vi "GUI.vi"() -> ()   [LabVIEW 2016]
uses:
  <vilib>/NI/Current Value Table/Type Defs/File Format.ctl
  <vilib>/NI/Current Value Table/Type Defs/Single Tag.ctl
  <vilib>/NI/Current Value Table/Type Defs/Data Types.ctl
  <vilib>/NI/Current Value Table/Type Defs/Tag Grouping set.ctl
  <vilib>/NI/Current Value Table/DataTypes/Boolean_Write.vi
  <vilib>/NI/Current Value Table/DataTypes/Boolean_Read.vi
  <vilib>/NI/Current Value Table/DataTypes/U16_Read.vi
  <vilib>/NI/Current Value Table/DataTypes/U16_Write.vi
  <vilib>/NI/Current Value Table/Type to Enum.vi
  <vilib>/NI/Current Value Table/DataTypes/Boolean_Type To Enum.vi
  <vilib>/NI/Current Value Table/DataTypes/U16_Type To Enum.vi
  MB_Master_Serial.lvclass
  C:/Users/PRANAV/Desktop/Modbus_Scada_Main/Modbus_Scada/MB_Master/MB_Master.lvclass
  <vilib>/NI/Current Value Table/FGVs/CVT Globals.vi
  <vilib>/NI/Current Value Table/FGVs/Tag Memory.vi
  <vilib>/NI/Current Value Table/Memory Block.vi
  <vilib>/NI/Current Value Table/DataTypes/Boolean_Memory Block.vi
  <vilib>/NI/Current Value Table/DataTypes/U16_Memory Block.vi
  <vilib>/NI/Current Value Table/Current Value Table.lvlib
  MB Master.lvlib
panel:
  out "Value_O2 3":u16
  out "Value_N2 3":u16
  out "Vel_Value 3":u16
  out "N2 Gas Pressure 1_Value 3":u16
  out "Temp_Min 4":u16
  out "Hum_Value  3":u16
  out "Value_O2 2":u16
  out "Value_N2 2":u16
  out "Vel_Value 2":u16
  out "N2 Gas Pressure 1_Value 2":u16
  out "Temp_Min 3":u16
  out "Hum_Value  2":u16
  out "Max_O2 2":u16
  out "Max_N2 2":u16
  out "Vel_Max 2":u16
  out "N2 Gas Pressure 1_Max 2":u16
  out "Temp_Max 2":u16
  out "Hum_Max 2":u16
  out "Min_O2 2":u16
  out "Min_N2 2":u16
  out "Vel_Min 2":u16
  out "N2 Gas Pressure 1_Min 2":u16
  out "Temp_Min 5":u16
  out "Hum_Min 2":u16
  out "Value_O2":u16
  out "Value_N2":u16
  out "Vel_Value":u16
  out "N2 Gas Pressure 1_Value":u16
  out "Temp_Min":u16
  out "Hum_Value":u16
  out "Spare AI-1_Value":u16
  out "Spare AI-2_Value":u16
  out "Max_O2":u16
  out "Max_N2":u16
  out "Vel_Max":u16
  out "N2 Gas Pressure 1_Max":u16
  out "Temp_Max":u16
  out "Hum_Max":u16
  out "Spare AI-1_Max":u16
  out "Spare AI-2_Max":u16
  out "Min_O2":u16
  out "Min_N2":u16
  out "Vel_Min":u16
  out "N2 Gas Pressure 1_Min":u16
  out "Temp_Min 2":u16
  out "Hum_Min":u16
  out "Spare AI-1_Min":u16
  out "Spare AI-2_Min":u16
  out "Value_8":bool
  out "Value_9":bool
  out "Value_10":bool
  out "Value_11":bool
  out "Value_12":bool
  out "Value_13":bool
  out "Value_14":bool
  out "Value_1":bool
  out "Value_2":bool
  out "Value_3":bool
  out "Value_4":bool
  out "Value_5":bool
  out "Value_6":bool
  out "Value_7":bool
  out "O.T. Entrance -Cap Proxy":bool
  out "Main Entrance E-stop PB":bool
  out "Doctors Entrance Door-2 Open Proxy FB":bool
  out "Main Entrance Door Open Inside PB":bool
  out "Main Entrance Door Open Proxy FB":bool
  out "O.T Entrance-Nose Mask Proxy":bool
  out "Doctors Entrance Door-1 Open PB":bool
  out "Doctors Entrance Door-1 Open Inside PB":bool
  out "Doctors Entrance Door-1 Open Proxy FB":bool
  out "Doctors Entrance-Nose Mask Proxy":bool
  out "Doctors Entrance-Cap Proxy":bool
  out "Doctors Entrance-Hand Sanitizer  Proxy":bool
  out "Doctors Entrance Door-2 Open Inside PB":bool
  out "Ist O.T.-Occupied Lamp Green":bool
  out "Ist O.T-AHU Start Coil":bool
  out "2nd O.T.:Scrubber Dispense Coil":bool
  out "2nd O.T.-Door Open Cmd":bool
  out "Spare DO-1":bool
  out "Spare DO-2":bool
  out "Spare DO-3":bool
  out "Spare DO-4":bool
  out "Spare DO-5":bool
  out "Spare DO-6":bool
  out "Doctor Entrance Door-1 Open Cmd":bool
  out "Doctor Entrance -Door-2 Open Cmd":bool
  out "Doctor Entrance -Hand Santizier Coil":bool
  out "Main Entrance-Door Open Cmd":bool
  out "OT Entrance-Door Open  Cmd":bool
  out "O.T Entrance-Hand Santiizier Coil":bool
  out "Ist O.T.- Door Open Cmd":bool
  out "Ist O.T-Occupied Lamp(Red)":bool
  out "Ist O.T-Inside Light":bool
  out "Ist O.T.-Scrubber Dispense Coil":bool
  out "error out":errorcluster
  in  "stop  5":bool
  in  "stop  4":bool
  in  "stop  3":bool
  in  "stop  2":bool
  in  "stop":bool
  # "DOORS &\n                    STATUS"
  # "Description"
  # "Status"
  # "Description"
  # "Status"
  # "Doctor Entrance Door-1 Open Cmd"
  # "Ist O.T.-Occupied Lamp Green"
  # "Doctor Entrance -Door-2 Open Cmd"
  # "Ist O.T-AHU Start Coil"
  # "Doctor Entrance -Hand Santizier Coil"
  # "2nd O.T.:Scrubber Dispense Coil"
  # "Main Entrance-Door Open Cmd"
  # "2nd O.T.-Door Open Cmd"
  # "OT Entrance-Door Open  Cmd"
  # "Spare DO-1"
  # "O.T Entrance-Hand Santiizier Coil"
  # "Spare DO-2"
  # "Ist O.T.- Door Open Cmd"
  # "Spare DO-3"
  # "Ist O.T-Occupied Lamp(Red)"
  # "Spare DO-4"
  # "Ist O.T-Inside Light"
  # "Spare DO-5"
  # "Ist O.T.-Scrubber Dispense Coil"
  # "Spare DO-6"
  # "DOORS FB AND SENSOR\n                                  STATUS"
  # "Description"
  # "Status"
  # "Description"
  # "Status"
  # "Doctors Entrance Door-1 Open PB"
  # "Doctors Entrance Door-2 Open Proxy FB"
  # "Doctors Entrance Door-1 Open Inside PB"
  # "Main Entrance E-stop PB"
  # "Doctors Entrance Door-1 Open Proxy FB"
  # "Main Entrance-Strecther Entry PB"
  # "Doctors Entrance-Nose Mask Proxy"
  # "Main Entrance Door Open Inside PB"
  # "Doctors Entrance-Cap Proxy"
  # "Main Entrance Door Open Proxy FB"
  # "Doctors Entrance-Hand Sanitizer  Proxy"
  # "O.T Entrance-Nose Mask Proxy"
  # "Doctors Entrance Door-2 Open Inside PB"
  # "O.T. Entrance -Cap Proxy"
  # "DOORS FB AND SENSOR\n                                  STATUS"
  # "Description"
  # "Status"
  # "Description"
  # "Status"
  # "OT Entrance-Hand Santizier Proxy"
  # "Spare DI-2"
  # "Spare DI-1"
  # "Ist O.T-AHU Run FB"
  # "OT Entrance-Door Inside Open PB"
  # "2nd O.T-Scrubber Proxy"
  # "OT Entrance-Door Open Proxy FB"
  # "2nd O.T-Door Inside Open PB"
  # "Ist O.T -Scrubber Proxy"
  # "2nd O.T-Door Open Proxy FB"
  # "Ist O.T-Door Inside Open PB"
  # "Ist O.T-E-Stop PB"
  # "Ist O.T-Door  Open Proxy FB"
  # "2nd O.T-E-Stop PB"
  # "O.T Parameters"
  # "Description"
  # "Min"
  # "Max"
  # "Value"
  # "Unit"
  # "O2 Gas Pressure"
  # "Bar"
  # "N2 Gas Pressure 1"
  # "Bar"
  # "Velocity"
  # "ft/m"
  # "N2 Gas Pressure 2"
  # "Bar"
  # "Room Temperature"
  # "Degree C"
  # "Relative Humidity"
  # "%"
  # "Spare AI 01"
  # "Spare AI 02"
  # "O.T Parameters S.P"
  # "Description"
  # "Very Low"
  # "Low"
  # "High"
  # "Very High"
  # "Unit"
  # "O2 Gas Pressure"
  # "Bar"
  # "N2 Gas Pressure 1"
  # "Bar"
  # "Velocity"
  # "ft/m"
  # "N2 Gas Pressure 2"
  # "Bar"
  # "Room Temperature"
  # "Degree C"
  # "Relative Humidity"
  # "%"
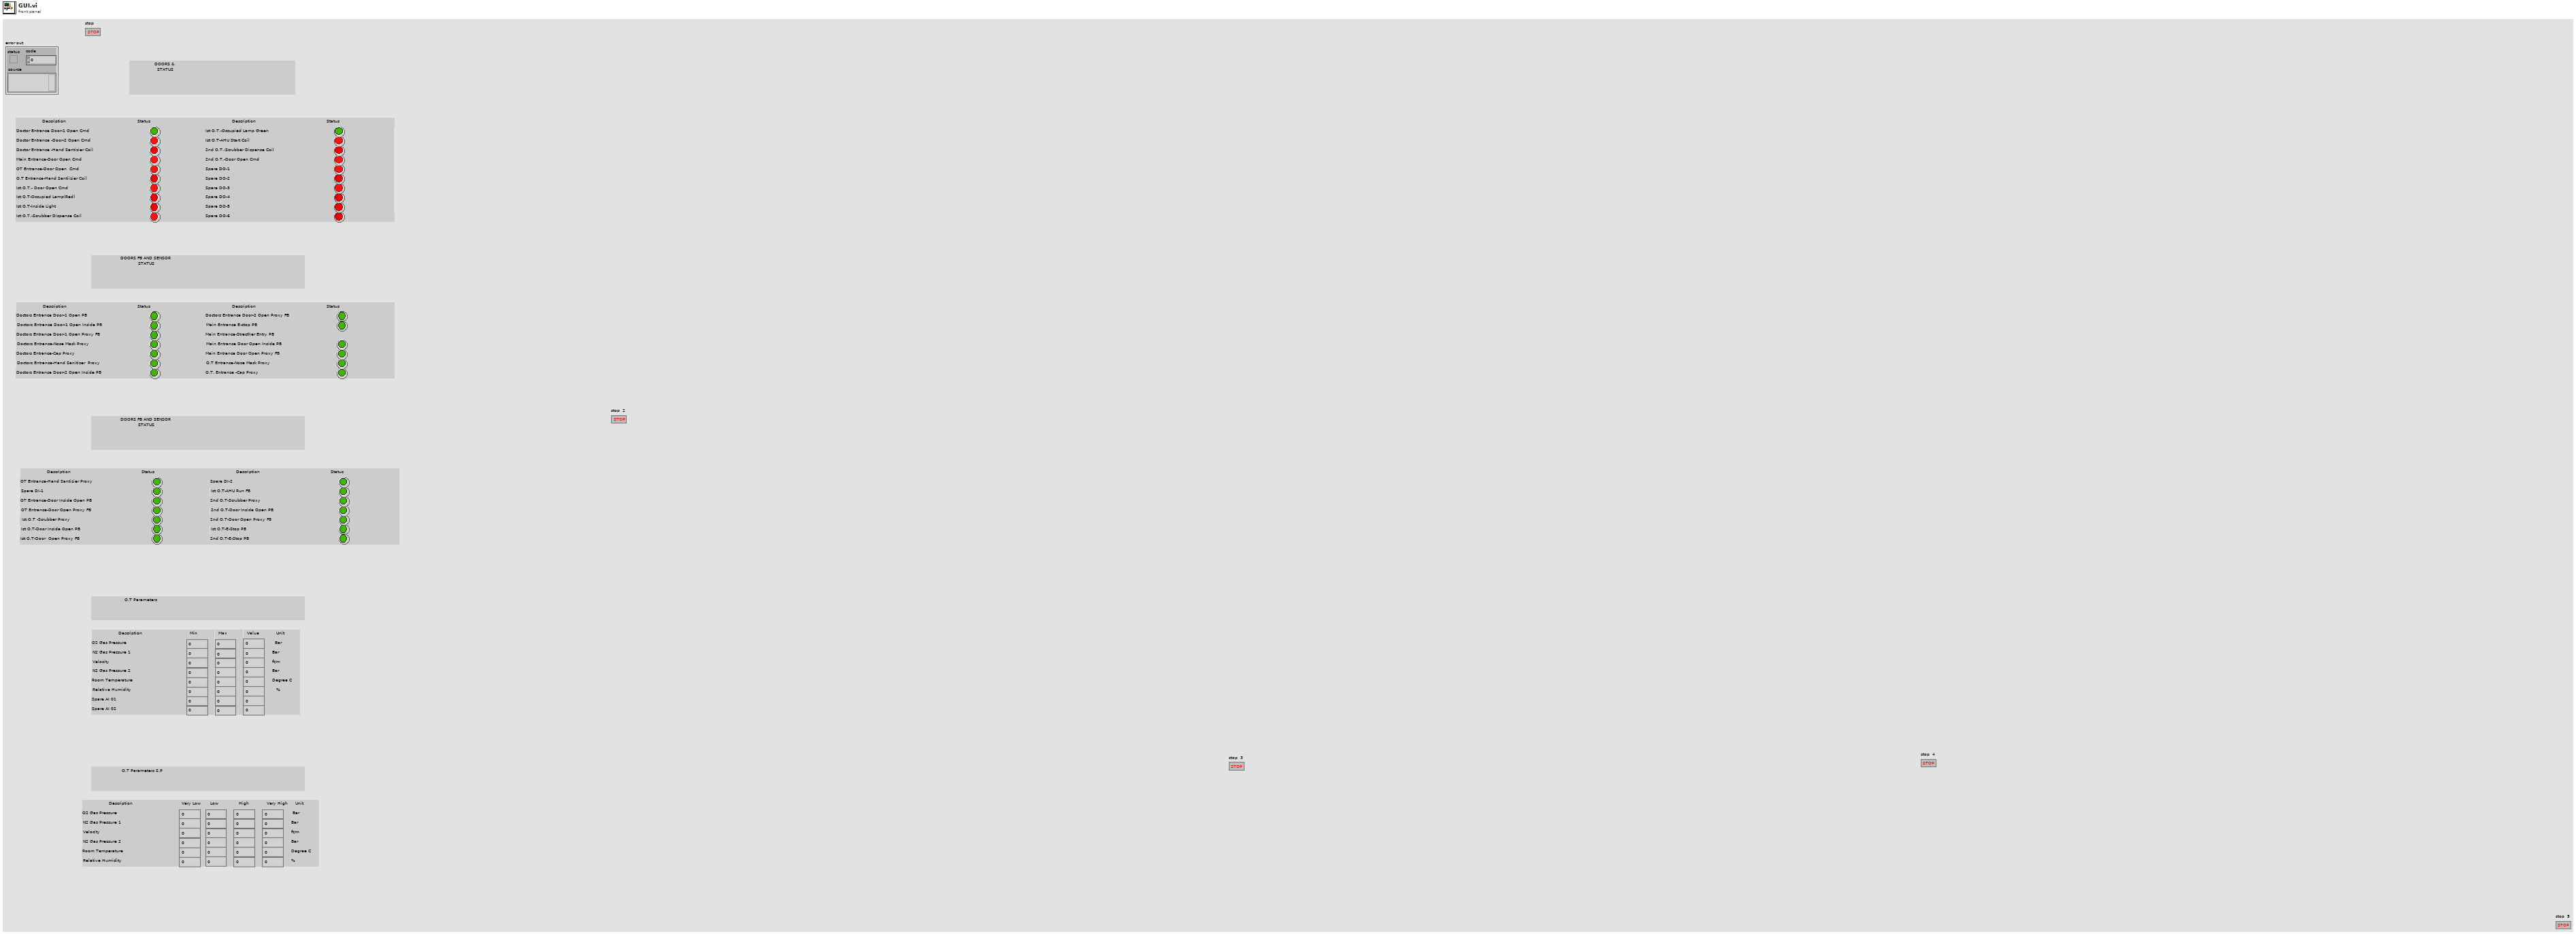
[diagram p1: front panel]
types:
  T1 = typedef "Current Value Table.lvlib/File Format.ctl" = cluster{"Tags":T2[], "Group Listings":T4[]}
  T2 = typedef "Current Value Table.lvlib/Single Tag.ctl" = cluster{"Data Type":T3, "Name":string, "Value":string, "Description":string}
  T3 = typedef "Current Value Table.lvlib/Data Types.ctl" = enum16{"Double", "Single", "I64", "I32", "I16", "I8", "U64", "U32", "U16", "U8", "String", "Boolean", "Array of U8", "Array of U16", "Array of U32", "Array of U64", "Array of I64", "Array of I32", "Array of I16", "Array of I8", "Array of Double", "Array of Single", "Array of Boolean", "Array of String"}
  T4 = typedef "Current Value Table.lvlib/Tag Grouping set.ctl" = cluster{"Group":string, "Tag Names":string[]}
  T5 = cluster{"baud rate (bps)":u32, "stop bits":u16, "parity":u16, "flow control":u16, "timeout":u32, "retries":i32}
diagram:
  n1 = call <vilib>:"Create Tags.vi"("Clear Table? (F)"=FALSE, "CVT Tags to Create"=T1 {"Tags"=[{"Data Type"=enum."Boolean", "Name"="Doctor Entrance Door-1 Open Cmd", "Value"="", "Description"=""}, {"Data Type"=enum."Boolean", "Name"="Doctor Entrance -Door-2 Open Cmd", "Value"="", "Description"=""}, {"Data Type"=enum."Boolean", "Name"="Doctor Entrance -Hand Santizier Coil", "Value"="", "Description"=""}, {"Data Type"=enum."Boolean", "Name"="Main Entrance-Door Open Cmd", "Value"="", "Description"=""}, {"Data Type"=enum."Boolean", "Name"="OT Entrance-Door Open  Cmd", "Value"="", "Description"=""}, {"Data Type"=enum."Boolean", "Name"="O.T Entrance-Hand Santiizier Coil", "Value"="", "Description"=""}, {"Data Type"=enum."Boolean", "Name"="Ist O.T.- Door Open Cmd", "Value"="", "Description"=""}, {"Data Type"=enum."Boolean", "Name"="Ist O.T-Occupied Lamp(Red)", "Value"="", "Description"=""}, {"Data Type"=enum."Boolean", "Name"="Ist O.T-Inside Light", "Value"="", "Description"=""}, {"Data Type"=enum."Boolean", "Name"="Ist O.T.-Scrubber Dispense Coil", "Value"="", "Description"=""}, {"Data Type"=enum."Boolean", "Name"="Ist O.T.-Occupied Lamp Green", "Value"="", "Description"=""}, {"Data Type"=enum."Boolean", "Name"="Ist O.T-AHU Start Coil", "Value"="", "Description"=""}, {"Data Type"=enum."Boolean", "Name"="2nd O.T.:Scrubber Dispense Coil", "Value"="", "Description"=""}, {"Data Type"=enum."Boolean", "Name"="2nd O.T.-Door Open Cmd", "Value"="", "Description"=""}, {"Data Type"=enum."Boolean", "Name"="Spare DO-1", "Value"="", "Description"=""}, {"Data Type"=enum."Boolean", "Name"="Spare DO-2", "Value"="", "Description"=""}, {"Data Type"=enum."Boolean", "Name"="Spare DO-3", "Value"="", "Description"=""}, {"Data Type"=enum."Boolean", "Name"="Spare DO-4", "Value"="", "Description"=""}, {"Data Type"=enum."Boolean", "Name"="Spare DO-5", "Value"="", "Description"=""}, {"Data Type"=enum."Boolean", "Name"="Spare DO-6", "Value"="", "Description"=""}, {"Data Type"=enum."Boolean", "Name"="Doctors Entrance Door-1 Open PB ", "Value"="", "Description"=""}, {"Data Type"=enum."Boolean", "Name"="Doctors Entrance Door-1 Open Inside PB", "Value"="", "Description"=""}, {"Data Type"=enum."Boolean", "Name"="Doctors Entrance Door-1 Open Proxy FB", "Value"="", "Description"=""}, {"Data Type"=enum."Boolean", "Name"="Doctors Entrance-Nose Mask Proxy", "Value"="", "Description"=""}, {"Data Type"=enum."Boolean", "Name"="Doctors Entrance-Cap Proxy", "Value"="", "Description"=""}, {"Data Type"=enum."Boolean", "Name"="Doctors Entrance-Hand Sanitizer  Proxy", "Value"="", "Description"=""}, {"Data Type"=enum."Boolean", "Name"="Doctors Entrance Door-2 Open Inside PB", "Value"="", "Description"=""}, {"Data Type"=enum."Boolean", "Name"="Doctors Entrance Door-2 Open Proxy FB ", "Value"="", "Description"=""}, {"Data Type"=enum."Boolean", "Name"="Main Entrance E-stop PB", "Value"="", "Description"=""}, {"Data Type"=enum."Boolean", "Name"="Main Entrance-Strecther Entry PB ", "Value"="", "Description"=""}, {"Data Type"=enum."Boolean", "Name"="Main Entrance Door Open Inside PB", "Value"="", "Description"=""}, {"Data Type"=enum."Boolean", "Name"="Main Entrance Door Open Proxy FB", "Value"="", "Description"=""}, {"Data Type"=enum."Boolean", "Name"="O.T Entrance-Nose Mask Proxy ", "Value"="", "Description"=""}, {"Data Type"=enum."Boolean", "Name"="O.T. Entrance -Cap Proxy", "Value"="", "Description"=""}, {"Data Type"=enum."Boolean", "Name"="OT Entrance-Hand Santizier Proxy", "Value"="", "Description"=""}, {"Data Type"=enum."Boolean", "Name"="Spare DI-1", "Value"="", "Description"=""}, {"Data Type"=enum."Boolean", "Name"="OT Entrance-Door Inside Open PB ", "Value"="", "Description"=""}, {"Data Type"=enum."Boolean", "Name"="OT Entrance-Door Open Proxy FB ", "Value"="", "Description"=""}, {"Data Type"=enum."Boolean", "Name"="Ist O.T -Scrubber Proxy", "Value"="", "Description"=""}, {"Data Type"=enum."Boolean", "Name"="Ist O.T-Door Inside Open PB", "Value"="", "Description"=""}, {"Data Type"=enum."Boolean", "Name"="Ist O.T-Door  Open Proxy FB ", "Value"="", "Description"=""}, {"Data Type"=enum."Boolean", "Name"="Spare DI-2", "Value"="", "Description"=""}, {"Data Type"=enum."Boolean", "Name"="Ist O.T-AHU Run FB", "Value"="", "Description"=""}, {"Data Type"=enum."Boolean", "Name"="2nd O.T-Scrubber Proxy", "Value"="", "Description"=""}, {"Data Type"=enum."Boolean", "Name"="2nd O.T-Door Inside Open PB", "Value"="", "Description"=""}, {"Data Type"=enum."Boolean", "Name"="2nd O.T-Door Open Proxy FB ", "Value"="", "Description"=""}, {"Data Type"=enum."Boolean", "Name"="Ist O.T-E-Stop PB", "Value"="", "Description"=""}, {"Data Type"=enum."Boolean", "Name"="2nd O.T-E-Stop PB ", "Value"="", "Description"=""}, {"Data Type"=enum."U16", "Name"="O2 Gas Pressure_Min", "Value"="", "Description"=""}, {"Data Type"=enum."Double", "Name"="O2 Gas Pressure", "Value"="", "Description"=""}, {"Data Type"=enum."U16", "Name"="O2 Gas Pressure _Value", "Value"="", "Description"=""}, {"Data Type"=enum."U16", "Name"="O2 Gas Pressure_Max", "Value"="", "Description"=""}, {"Data Type"=enum."U16", "Name"="N2 Gas Pressure_Min", "Value"="", "Description"=""}, {"Data Type"=enum."U16", "Name"="N2 Gas Pressure_Max", "Value"="", "Description"=""}, {"Data Type"=enum."U16", "Name"="N2 Gas Pressure_Value", "Value"="", "Description"=""}, {"Data Type"=enum."U16", "Name"="Velocity_Min", "Value"="", "Description"=""}, {"Data Type"=enum."U16", "Name"="Velocity_Max", "Value"="", "Description"=""}, {"Data Type"=enum."U16", "Name"="Velocity_Value", "Value"="", "Description"=""}, {"Data Type"=enum."U16", "Name"="N2 Gas Pressure 1_Min", "Value"="", "Description"=""}, {"Data Type"=enum."U16", "Name"="N2 Gas Pressure 1 _Max", "Value"="", "Description"=""}, {"Data Type"=enum."U16", "Name"="N2 Gas Pressure 1_Value", "Value"="", "Description"=""}, {"Data Type"=enum."U16", "Name"="Temp_Min", "Value"="", "Description"=""}, {"Data Type"=enum."U16", "Name"="Temp_Max", "Value"="", "Description"=""}, {"Data Type"=enum."U16", "Name"="Temp_Value", "Value"="", "Description"=""}, {"Data Type"=enum."U16", "Name"="Hum_Min", "Value"="", "Description"=""}, {"Data Type"=enum."U16", "Name"="Hum_Max", "Value"="", "Description"=""}, {"Data Type"=enum."U16", "Name"="Hum_Value", "Value"="", "Description"=""}, {"Data Type"=enum."U16", "Name"="Spare AI-1_Min", "Value"="", "Description"=""}, {"Data Type"=enum."U16", "Name"="Spare AI-1_Max", "Value"="", "Description"=""}, {"Data Type"=enum."U16", "Name"="Spare AI-1_Value", "Value"="", "Description"=""}, {"Data Type"=enum."U16", "Name"="Spare AI-2_Min", "Value"="", "Description"=""}, {"Data Type"=enum."U16", "Name"="Spare AI-2_Max", "Value"="", "Description"=""}, {"Data Type"=enum."U16", "Name"="Spare AI-2_Value", "Value"="", "Description"=""}, {"Data Type"=enum."Boolean", "Name"="Value_1", "Value"="", "Description"=""}, {"Data Type"=enum."Boolean", "Name"="Value_2", "Value"="", "Description"=""}, {"Data Type"=enum."Boolean", "Name"="Value_3", "Value"="", "Description"=""}, {"Data Type"=enum."Boolean", "Name"="Value_4", "Value"="", "Description"=""}, {"Data Type"=enum."Boolean", "Name"="Value_5", "Value"="", "Description"=""}, {"Data Type"=enum."Boolean", "Name"="Value_6", "Value"="", "Description"=""}, {"Data Type"=enum."Boolean", "Name"="Value_7", "Value"="", "Description"=""}, {"Data Type"=enum."Boolean", "Name"="Value_8", "Value"="", "Description"=""}, {"Data Type"=enum."Boolean", "Name"="Value_9", "Value"="", "Description"=""}, {"Data Type"=enum."Boolean", "Name"="Value_10", "Value"="", "Description"=""}, {"Data Type"=enum."Boolean", "Name"="Value_11", "Value"="", "Description"=""}, {"Data Type"=enum."Boolean", "Name"="Value_12", "Value"="", "Description"=""}, {"Data Type"=enum."Boolean", "Name"="Value_13", "Value"="", "Description"=""}, {"Data Type"=enum."Boolean", "Name"="Value_14", "Value"="", "Description"=""}, {"Data Type"=enum."U16", "Name"="O2_L1", "Value"="", "Description"=""}, {"Data Type"=enum."U16", "Name"="O2_L2", "Value"="", "Description"=""}, {"Data Type"=enum."U16", "Name"="O2_H1", "Value"="", "Description"=""}, {"Data Type"=enum."U16", "Name"="O2_H2", "Value"="", "Description"=""}, {"Data Type"=enum."U16", "Name"="N21_L1", "Value"="", "Description"=""}, {"Data Type"=enum."U16", "Name"="N21_L2", "Value"="", "Description"=""}, {"Data Type"=enum."U16", "Name"="N21_H1", "Value"="", "Description"=""}, {"Data Type"=enum."U16", "Name"="N21_H2", "Value"="", "Description"=""}, {"Data Type"=enum."U16", "Name"="Vel_L1", "Value"="", "Description"=""}, {"Data Type"=enum."U16", "Name"="Vel_L2", "Value"="", "Description"=""}, {"Data Type"=enum."U16", "Name"="Vel_H1", "Value"="", "Description"=""}, {"Data Type"=enum."U16", "Name"="Vel_H2", "Value"="", "Description"=""}, {"Data Type"=enum."U16", "Name"="N22_L1", "Value"="", "Description"=""}, {"Data Type"=enum."U16", "Name"="N22_L2", "Value"="", "Description"=""}, {"Data Type"=enum."U16", "Name"="N22_H1", "Value"="", "Description"=""}, {"Data Type"=enum."U16", "Name"="N22_H2", "Value"="", "Description"=""}, {"Data Type"=enum."U16", "Name"="Temp_L1", "Value"="", "Description"=""}, {"Data Type"=enum."U16", "Name"="Temp_L2", "Value"="", "Description"=""}, {"Data Type"=enum."U16", "Name"="Temp_H1", "Value"="", "Description"=""}, {"Data Type"=enum."U16", "Name"="Temp_H2", "Value"="", "Description"=""}, {"Data Type"=enum."U16", "Name"="RH_L1", "Value"="", "Description"=""}, {"Data Type"=enum."U16", "Name"="RH_L2", "Value"="", "Description"=""}, {"Data Type"=enum."U16", "Name"="RH_H1", "Value"="", "Description"=""}, {"Data Type"=enum."U16", "Name"="RH_H2", "Value"="", "Description"=""}], "Group Listings"=[]}) -> ("error out"=w6:errorcluster)  [unwired: 9 in]
  n2 = call "Open Serial Session.vi"("Error in"=w6, "Slave ID"=u8 5, "Serial Config"=T5 {"baud rate (bps)"=19200, "stop bits"=10, "parity"=0, "flow control"=0, "timeout"=10000, "retries"=1}, "VISA Resource"=refnum<visa-resource-name> "COM6") -> ("Error out"=w4:errorcluster, "MB_Serial session"=w5:refnum<class "MB_Master_Serial.lvclass">)  [unwired: 6 in]
  n3 = while {
    shift-right: [w27] -> w3
    shift-left: w5 -> [w28]
    shift-right: [w26] -> w2
    shift-left: w4 -> [w29]
    stop <- w12 stop-if-true
    n4 = flat-sequence {
      tunnel: w29 -> [w31]
      tunnel: w28 -> [w32]
      tunnel: [w156] -> w25
      tunnel: [w38] -> w24
      tunnel: [w34] -> w23
      tunnel: [w30] -> w22
      tunnel: w25 -> [_]
      tunnel: w24 -> [w165]
      tunnel: w23 -> [_]
      tunnel: w22 -> [w166]
      tunnel: [w235] -> w21
      tunnel: [w161] -> w20
      tunnel: [w160] -> w19
      tunnel: w21 -> [_]
      tunnel: w20 -> [w253]
      tunnel: w19 -> [w254]
      tunnel: [w388] -> w18
      tunnel: [w249] -> w17
      tunnel: [w250] -> w16
      tunnel: w18 -> [_]
      tunnel: w17 -> [w409]
      tunnel: w16 -> [w412]
      tunnel: [w408] -> w15
      tunnel: [w410] -> w14
      tunnel: [w492] -> w13
      tunnel: [w503] -> w27
      tunnel: [w504] -> w26
      tunnel: w15 -> [w505]
      tunnel: w14 -> [w501]
      tunnel: w13 -> [_]
      tunnel: [w624] -> w12
      frame #0 {
        w43 = "Spare DO-6" ("Tag Name")
        w50 = "Spare DO-5" ("Tag Name")
        w54 = "Spare DO-4" ("Tag Name")
        w58 = "Spare DO-3" ("Tag Name")
        w64 = "Spare DO-2" ("Tag Name")
        w37 = "Spare DO-1" ("Tag Name")
        w77 = "2nd O.T.-Door Open Cmd" ("Tag Name")
        w82 = "2nd O.T.:Scrubber Dispense Coil" ("Tag Name")
        w89 = "Ist O.T-AHU Start Coil" ("Tag Name")
        w92 = "Ist O.T.-Occupied Lamp Green" ("Tag Name")
        w101 = "Ist O.T.-Scrubber Dispense Coil" ("Tag Name")
        w105 = "Ist O.T-Inside Light" ("Tag Name")
        w113 = "Ist O.T-Occupied Lamp(Red)" ("Tag Name")
        w118 = "Ist O.T.- Door Open Cmd" ("Tag Name")
        w123 = "O.T Entrance-Hand Santiizier Coil" ("Tag Name")
        w141 = "OT Entrance-Door Open  Cmd" ("Tag Name")
        w144 = "Main Entrance-Door Open Cmd" ("Tag Name")
        w147 = "Doctor Entrance -Hand Santizier Coil" ("Tag Name")
        w153 = "Doctor Entrance -Door-2 Open Cmd" ("Tag Name")
        w159 = "Doctor Entrance Door-1 Open Cmd" ("Tag Name")
        n5 = call "Read Coils.vi"("error in (no error)"=w31, "quantity"=u16 22, "starting address"=u16 0, "MB session in"=w32) -> ("error out"=w33:errorcluster, "Coils"=w34:bool[], "MB session out"=w30:refnum<class "MB_Master_Serial.lvclass">)  [unwired: 5 in]
        n6 = Index Array(array=w34, index #1=0 ("index"), index #2=1 ("index"), index #3=2 ("index"), index #4=3 ("index"), index #5=4 ("index"), index #6=5 ("index"), index #7=6 ("index"), index #8=7 ("index"), index #9=8 ("index"), index #10=9 ("index"), index #11=10 ("index"), index #12=11 ("index"), index #13=12 ("index"), index #14=13 ("index"), index #15=14 ("index"), index #16=15 ("index"), index #17=16 ("index"), index #18=17 ("index"), index #19=18 ("index"), index #20=19 ("index")) -> (element #1=w136:bool, element #2=w134:bool, element #3=w132:bool, element #4=w130:bool, element #5=w128:bool, element #6=w126:bool, element #7=w120:bool, element #8=w114:bool, element #9=w108:bool, element #10=w102:bool, element #11=w96:bool, element #12=w90:bool, element #13=w84:bool, element #14=w78:bool, element #15=w71:bool, element #16=w66:bool, element #17=w61:bool, element #18=w55:bool, element #19=w51:bool, element #20=w42:bool)
        n7 = call-poly <vilib>:"Write.vi"("error in (no error)"=w33, "Value"=w136, "Tag Name"=w159) -> ("error out"=w152:errorcluster)  [unwired: 8 in]
        n8 = call-poly <vilib>:"Write.vi"("error in (no error)"=w152, "Value"=w134, "Tag Name"=w153) -> ("error out"=w149:errorcluster)  [unwired: 8 in]
        n9 = call-poly <vilib>:"Write.vi"("error in (no error)"=w149, "Value"=w132, "Tag Name"=w147) -> ("error out"=w145:errorcluster)  [unwired: 8 in]
        n10 = call-poly <vilib>:"Write.vi"("error in (no error)"=w145, "Value"=w130, "Tag Name"=w144) -> ("error out"=w138:errorcluster)  [unwired: 8 in]
        n11 = call-poly <vilib>:"Write.vi"("error in (no error)"=w138, "Value"=w128, "Tag Name"=w141) -> ("error out"=w125:errorcluster)  [unwired: 8 in]
        n12 = call-poly <vilib>:"Write.vi"("error in (no error)"=w125, "Value"=w126, "Tag Name"=w123) -> ("error out"=w119:errorcluster)  [unwired: 8 in]
        n13 = call-poly <vilib>:"Write.vi"("error in (no error)"=w119, "Value"=w120, "Tag Name"=w118) -> ("error out"=w112:errorcluster)  [unwired: 8 in]
        n14 = call-poly <vilib>:"Write.vi"("error in (no error)"=w112, "Value"=w114, "Tag Name"=w113) -> ("error out"=w107:errorcluster)  [unwired: 8 in]
        n15 = call-poly <vilib>:"Write.vi"("error in (no error)"=w107, "Value"=w108, "Tag Name"=w105) -> ("error out"=w100:errorcluster)  [unwired: 8 in]
        n16 = call-poly <vilib>:"Write.vi"("error in (no error)"=w100, "Value"=w102, "Tag Name"=w101) -> ("error out"=w93:errorcluster)  [unwired: 8 in]
        n17 = call-poly <vilib>:"Write.vi"("error in (no error)"=w93, "Value"=w96, "Tag Name"=w92) -> ("error out"=w88:errorcluster)  [unwired: 8 in]
        n18 = call-poly <vilib>:"Write.vi"("error in (no error)"=w88, "Value"=w90, "Tag Name"=w89) -> ("error out"=w83:errorcluster)  [unwired: 8 in]
        n19 = call-poly <vilib>:"Write.vi"("error in (no error)"=w83, "Value"=w84, "Tag Name"=w82) -> ("error out"=w76:errorcluster)  [unwired: 8 in]
        n20 = call-poly <vilib>:"Write.vi"("error in (no error)"=w76, "Value"=w78, "Tag Name"=w77) -> ("error out"=w73:errorcluster)  [unwired: 8 in]
        n21 = call-poly <vilib>:"Write.vi"("error in (no error)"=w73, "Value"=w71, "Tag Name"=w37) -> ("error out"=w68:errorcluster)  [unwired: 8 in]
        n22 = call-poly <vilib>:"Write.vi"("error in (no error)"=w68, "Value"=w66, "Tag Name"=w64) -> ("error out"=w60:errorcluster)  [unwired: 8 in]
        n23 = call-poly <vilib>:"Write.vi"("error in (no error)"=w60, "Value"=w61, "Tag Name"=w58) -> ("error out"=w48:errorcluster)  [unwired: 8 in]
        n24 = call-poly <vilib>:"Write.vi"("error in (no error)"=w48, "Value"=w55, "Tag Name"=w54) -> ("error out"=w49:errorcluster)  [unwired: 8 in]
        n25 = call-poly <vilib>:"Write.vi"("error in (no error)"=w49, "Value"=w51, "Tag Name"=w50) -> ("error out"=w41:errorcluster)  [unwired: 8 in]
        n26 = call-poly <vilib>:"Write.vi"("error in (no error)"=w41, "Value"=w42, "Tag Name"=w43) -> ()  [unwired: 8 in, 1 out]
        n27 = call-poly <vilib>:"Read.vi"("error in (no error)"=w152, "Tag Name"=w159) -> ("error out"=w151:errorcluster, "Value"=→"Doctor Entrance Door-1 Open Cmd":bool)  [unwired: 8 in]
        n28 = call-poly <vilib>:"Read.vi"("error in (no error)"=w151, "Tag Name"=w153) -> ("error out"=w148:errorcluster, "Value"=→"Doctor Entrance -Door-2 Open Cmd":bool)  [unwired: 8 in]
        n29 = call-poly <vilib>:"Read.vi"("error in (no error)"=w148, "Tag Name"=w147) -> ("error out"=w143:errorcluster, "Value"=→"Doctor Entrance -Hand Santizier Coil":bool)  [unwired: 8 in]
        n30 = Wait (ms)(milliseconds to wait=u32 500) -> ()  [unwired: 1 out]
        n31 = call-poly <vilib>:"Read.vi"("error in (no error)"=w143, "Tag Name"=w144) -> ("error out"=w140:errorcluster, "Value"=→"Main Entrance-Door Open Cmd":bool)  [unwired: 8 in]
        n32 = call-poly <vilib>:"Read.vi"("error in (no error)"=w140, "Tag Name"=w141) -> ("error out"=w124:errorcluster, "Value"=→"OT Entrance-Door Open  Cmd":bool)  [unwired: 8 in]
        n33 = call-poly <vilib>:"Read.vi"("error in (no error)"=w124, "Tag Name"=w123) -> ("error out"=w117:errorcluster, "Value"=→"O.T Entrance-Hand Santiizier Coil":bool)  [unwired: 8 in]
        n34 = call-poly <vilib>:"Read.vi"("error in (no error)"=w117, "Tag Name"=w118) -> ("error out"=w111:errorcluster, "Value"=→"Ist O.T.- Door Open Cmd":bool)  [unwired: 8 in]
        n35 = call-poly <vilib>:"Read.vi"("error in (no error)"=w111, "Tag Name"=w113) -> ("error out"=w106:errorcluster, "Value"=→"Ist O.T-Occupied Lamp(Red)":bool)  [unwired: 8 in]
        n36 = call-poly <vilib>:"Read.vi"("error in (no error)"=w106, "Tag Name"=w105) -> ("error out"=w99:errorcluster, "Value"=→"Ist O.T-Inside Light":bool)  [unwired: 8 in]
        n37 = call-poly <vilib>:"Read.vi"("error in (no error)"=w99, "Tag Name"=w101) -> ("error out"=w94:errorcluster, "Value"=→"Ist O.T.-Scrubber Dispense Coil":bool)  [unwired: 8 in]
        n38 = call-poly <vilib>:"Read.vi"("error in (no error)"=w94, "Tag Name"=w92) -> ("error out"=w87:errorcluster, "Value"=→"Ist O.T.-Occupied Lamp Green":bool)  [unwired: 8 in]
        n39 = call-poly <vilib>:"Read.vi"("error in (no error)"=w87, "Tag Name"=w89) -> ("error out"=w81:errorcluster, "Value"=→"Ist O.T-AHU Start Coil":bool)  [unwired: 8 in]
        n40 = call-poly <vilib>:"Read.vi"("error in (no error)"=w81, "Tag Name"=w82) -> ("error out"=w75:errorcluster, "Value"=→"2nd O.T.:Scrubber Dispense Coil":bool)  [unwired: 8 in]
        n41 = call-poly <vilib>:"Read.vi"("error in (no error)"=w75, "Tag Name"=w77) -> ("error out"=w70:errorcluster, "Value"=→"2nd O.T.-Door Open Cmd":bool)  [unwired: 8 in]
        n42 = call-poly <vilib>:"Read.vi"("error in (no error)"=w70, "Tag Name"=w37) -> ("error out"=w65:errorcluster, "Value"=→"Spare DO-1":bool)  [unwired: 8 in]
        n43 = call-poly <vilib>:"Read.vi"("error in (no error)"=w65, "Tag Name"=w64) -> ("error out"=w59:errorcluster, "Value"=→"Spare DO-2":bool)  [unwired: 8 in]
        n44 = call-poly <vilib>:"Read.vi"("error in (no error)"=w59, "Tag Name"=w58) -> ("error out"=w47:errorcluster, "Value"=→"Spare DO-3":bool)  [unwired: 8 in]
        n45 = call-poly <vilib>:"Read.vi"("error in (no error)"=w47, "Tag Name"=w54) -> ("error out"=w46:errorcluster, "Value"=→"Spare DO-4":bool)  [unwired: 8 in]
        n46 = call-poly <vilib>:"Read.vi"("error in (no error)"=w46, "Tag Name"=w50) -> ("error out"=w40:errorcluster, "Value"=→"Spare DO-5":bool)  [unwired: 8 in]
        n47 = call-poly <vilib>:"Read.vi"("error in (no error)"=w40, "Tag Name"=w43) -> ("error out"=w38:errorcluster, "Value"=→"Spare DO-6":bool)  [unwired: 8 in]
        n48 = Unbundle By Name(w38) -> ("status"=w157:bool)
        n49 = Or(x=w157, y="stop") -> (x .or. y?=w156:bool)
      }
      frame #1 {
        w173 = "O.T Entrance-Nose Mask Proxy " ("Tag Name")
        w178 = "Main Entrance Door Open Proxy FB" ("Tag Name")
        w183 = "Main Entrance Door Open Inside PB" ("Tag Name")
        w189 = "Doctors Entrance Door-2 Open Proxy FB " ("Tag Name")
        w195 = "Main Entrance E-stop PB" ("Tag Name")
        (unwired) FALSE ("Value")
        w201 = "O.T. Entrance -Cap Proxy" ("Tag Name")
        w209 = "Doctors Entrance Door-2 Open Inside PB" ("Tag Name")
        w212 = "Doctors Entrance-Hand Sanitizer  Proxy" ("Tag Name")
        w219 = "Doctors Entrance-Cap Proxy" ("Tag Name")
        w226 = "Doctors Entrance-Nose Mask Proxy" ("Tag Name")
        w232 = "Doctors Entrance Door-1 Open Proxy FB" ("Tag Name")
        w239 = "Doctors Entrance Door-1 Open Inside PB" ("Tag Name")
        w244 = "Doctors Entrance Door-1 Open PB " ("Tag Name")
        n50 = call "Read Discrete Inputs.vi"("error in (no error)"=w165, "quantity"=u16 16 ("Quantity"), "starting address"=u16 0 ("Starting Address"), "MB session in"=w166) -> ("error out"=w161:errorcluster, "Inputs"=w162:bool[], "MB session out"=w160:refnum<class "MB_Master_Serial.lvclass">)  [unwired: 5 in]
        n51 = Index Array(array=w162, index #1=0 ("index"), index #2=1 ("index"), index #3=2 ("index"), index #4=3 ("index"), index #5=4 ("index"), index #6=5 ("index"), index #7=6 ("index"), index #8=8 ("index"), index #9=9 ("index"), index #10=10 ("index"), index #11=11 ("index"), index #12=12 ("index"), index #13=13 ("index"), index #14=14 ("index")) -> (element #1=w247:bool, element #2=w240:bool, element #3=w233:bool, element #4=w227:bool, element #5=w221:bool, element #6=w213:bool, element #7=w207:bool, element #8=w203:bool, element #9=w197:bool, element #10=w190:bool, element #12=w184:bool, element #13=w180:bool, element #14=w174:bool)  [unwired: 1 out]
        n52 = call-poly <vilib>:"Write.vi"("Value"=w247, "Tag Name"=w244) -> ("error out"=w246:errorcluster)  [unwired: 9 in]
        n53 = call-poly <vilib>:"Write.vi"("error in (no error)"=w246, "Value"=w240, "Tag Name"=w239) -> ("error out"=w230:errorcluster)  [unwired: 8 in]
        n54 = call-poly <vilib>:"Write.vi"("error in (no error)"=w230, "Value"=w233, "Tag Name"=w232) -> ("error out"=w225:errorcluster)  [unwired: 8 in]
        n55 = call-poly <vilib>:"Write.vi"("error in (no error)"=w225, "Value"=w227, "Tag Name"=w226) -> ("error out"=w220:errorcluster)  [unwired: 8 in]
        n56 = call-poly <vilib>:"Write.vi"("error in (no error)"=w220, "Value"=w221, "Tag Name"=w219) -> ("error out"=w216:errorcluster)  [unwired: 8 in]
        n57 = call-poly <vilib>:"Write.vi"("error in (no error)"=w216, "Value"=w213, "Tag Name"=w212) -> ("error out"=w208:errorcluster)  [unwired: 8 in]
        n58 = call-poly <vilib>:"Write.vi"("error in (no error)"=w208, "Value"=w207, "Tag Name"=w209) -> ("error out"=w202:errorcluster)  [unwired: 8 in]
        n59 = call-poly <vilib>:"Write.vi"("error in (no error)"=w202, "Value"=w203, "Tag Name"=w201) -> ("error out"=w196:errorcluster)  [unwired: 8 in]
        n60 = call-poly <vilib>:"Write.vi"("error in (no error)"=w196, "Value"=w197, "Tag Name"=w195) -> ("error out"=w191:errorcluster)  [unwired: 8 in]
        n61 = call-poly <vilib>:"Write.vi"("error in (no error)"=w191, "Value"=w190, "Tag Name"=w189) -> ("error out"=w168:errorcluster)  [unwired: 8 in]
        n62 = call-poly <vilib>:"Write.vi"("error in (no error)"=w168, "Value"=w184, "Tag Name"=w183) -> ("error out"=w179:errorcluster)  [unwired: 8 in]
        n63 = call-poly <vilib>:"Write.vi"("error in (no error)"=w179, "Value"=w180, "Tag Name"=w178) -> ("error out"=w172:errorcluster)  [unwired: 8 in]
        n64 = call-poly <vilib>:"Write.vi"("error in (no error)"=w172, "Value"=w174, "Tag Name"=w173) -> ()  [unwired: 8 in, 1 out]
        n65 = call-poly <vilib>:"Read.vi"("error in (no error)"=w246, "Tag Name"=w244) -> ("error out"=w245:errorcluster, "Value"=→"Doctors Entrance Door-1 Open PB":bool)  [unwired: 8 in]
        n66 = call-poly <vilib>:"Read.vi"("error in (no error)"=w245, "Tag Name"=w239) -> ("error out"=w231:errorcluster, "Value"=→"Doctors Entrance Door-1 Open Inside PB":bool)  [unwired: 8 in]
        n67 = call-poly <vilib>:"Read.vi"("error in (no error)"=w231, "Tag Name"=w232) -> ("error out"=w224:errorcluster, "Value"=→"Doctors Entrance Door-1 Open Proxy FB":bool)  [unwired: 8 in]
        n68 = call-poly <vilib>:"Read.vi"("error in (no error)"=w224, "Tag Name"=w226) -> ("error out"=w218:errorcluster, "Value"=→"Doctors Entrance-Nose Mask Proxy":bool)  [unwired: 8 in]
        n69 = call-poly <vilib>:"Read.vi"("error in (no error)"=w218, "Tag Name"=w219) -> ("error out"=w215:errorcluster, "Value"=→"Doctors Entrance-Cap Proxy":bool)  [unwired: 8 in]
        n70 = call-poly <vilib>:"Read.vi"("error in (no error)"=w215, "Tag Name"=w212) -> ("error out"=w205:errorcluster, "Value"=→"Doctors Entrance-Hand Sanitizer  Proxy":bool)  [unwired: 8 in]
        n71 = call-poly <vilib>:"Read.vi"("error in (no error)"=w205, "Tag Name"=w209) -> ("error out"=w200:errorcluster, "Value"=→"Doctors Entrance Door-2 Open Inside PB":bool)  [unwired: 8 in]
        n72 = call-poly <vilib>:"Read.vi"("error in (no error)"=w200, "Tag Name"=w201) -> ("error out"=w194:errorcluster, "Value"=→"O.T. Entrance -Cap Proxy":bool)  [unwired: 8 in]
        n73 = call-poly <vilib>:"Read.vi"("error in (no error)"=w194, "Tag Name"=w195) -> ("error out"=w188:errorcluster, "Value"=→"Main Entrance E-stop PB":bool)  [unwired: 8 in]
        n74 = call-poly <vilib>:"Read.vi"("error in (no error)"=w188, "Tag Name"=w189) -> ("error out"=w167:errorcluster, "Value"=→"Doctors Entrance Door-2 Open Proxy FB":bool)  [unwired: 8 in]
        n75 = call-poly <vilib>:"Read.vi"("error in (no error)"=w167, "Tag Name"=w183) -> ("error out"=w177:errorcluster, "Value"=→"Main Entrance Door Open Inside PB":bool)  [unwired: 8 in]
        n76 = call-poly <vilib>:"Read.vi"("error in (no error)"=w177, "Tag Name"=w178) -> ("error out"=w171:errorcluster, "Value"=→"Main Entrance Door Open Proxy FB":bool)  [unwired: 8 in]
        n77 = call-poly <vilib>:"Read.vi"("error in (no error)"=w171, "Tag Name"=w173) -> ("error out"=w170:errorcluster, "Value"=→"O.T Entrance-Nose Mask Proxy":bool)  [unwired: 8 in]
        n78 = Unbundle By Name(w170) -> ("status"=w236:bool)
        n79 = Or(x=w236, y="stop  2") -> (x .or. y?=w235:bool)
      }
      frame #2 {
        w262 = "Spare AI-2_Min" ("Tag Name")
        w263 = "Spare AI-2_Value" ("Tag Name")
        w264 = "Spare AI-2_Max" ("Tag Name")
        w281 = "Spare AI-1_Value" ("Tag Name")
        w282 = "Spare AI-1_Max" ("Tag Name")
        w284 = "Spare AI-1_Min" ("Tag Name")
        w298 = "Hum_Value" ("Tag Name")
        w299 = "Hum_Max" ("Tag Name")
        w300 = "Hum_Min" ("Tag Name")
        w318 = "Temp_Value" ("Tag Name")
        w317 = "Temp_Max" ("Tag Name")
        w315 = "Temp_Min" ("Tag Name")
        w331 = "N2 Gas Pressure 1_Value" ("Tag Name")
        w336 = "N2 Gas Pressure 1 _Max" ("Tag Name")
        w337 = "N2 Gas Pressure 1_Min" ("Tag Name")
        w351 = "Velocity_Value" ("Tag Name")
        w353 = "Velocity_Max" ("Tag Name")
        w356 = "Velocity_Min" ("Tag Name")
        w371 = "N2 Gas Pressure_Value" ("Tag Name")
        w376 = "N2 Gas Pressure_Max" ("Tag Name")
        w380 = "N2 Gas Pressure_Min" ("Tag Name")
        w386 = "O2 Gas Pressure _Value" ("Tag Name")
        w387 = "O2 Gas Pressure_Max" ("Tag Name")
        w394 = "O2 Gas Pressure_Min" ("Tag Name")
        n80 = call "Read Input Registers.vi"("error in (no error)"=w253, "quantity"=u16 25 ("Starting Address"), "starting address"=u16 0 ("Starting Address"), "MB session in"=w254) -> ("error out"=w249:errorcluster, "Registers"=w248:u16[], "MB session out"=w250:refnum<class "MB_Master_Serial.lvclass">)  [unwired: 5 in]
        n81 = Index Array(array=w248, index #1=21 ("index"), index #2=22 ("index"), index #3=23 ("index")) -> (element #1=w267:u16, element #2=w266:u16, element #3=w265:u16)
        n82 = Index Array(array=w248, index #1=3 ("index"), index #2=4 ("index"), index #3=5 ("index")) -> (element #1=w382:u16, element #2=w377:u16, element #3=w369:u16)
        n83 = Index Array(array=w248, index #1=18 ("index"), index #2=19 ("index"), index #3=20 ("index")) -> (element #1=w287:u16, element #2=w286:u16, element #3=w285:u16)
        n84 = Index Array(array=w248, index #1=6 ("index"), index #2=7 ("index"), index #3=8 ("index")) -> (element #1=w361:u16, element #2=w360:u16, element #3=w359:u16)
        n85 = Index Array(array=w248, index #1=9 ("index"), index #2=10 ("index"), index #3=11 ("index")) -> (element #1=w344:u16, element #2=w343:u16, element #3=w342:u16)
        n86 = Index Array(array=w248, index #1=12 ("index"), index #2=13 ("index"), index #3=14 ("index")) -> (element #1=w326:u16, element #2=w325:u16, element #3=w324:u16)
        n87 = Index Array(array=w248, index #1=0 ("index"), index #2=1 ("index"), index #3=2 ("index")) -> (element #1=w404:u16, element #2=w402:u16, element #3=w396:u16)
        n88 = Index Array(array=w248, index #1=15 ("index"), index #2=16 ("index"), index #3=17 ("index")) -> (element #1=w303:u16, element #2=w302:u16, element #3=w301:u16)
        n89 = call-poly <vilib>:"Write.vi"("error in (no error)"=w249, "Value"=w404, "Tag Name"=w394) -> ("error out"=w401:errorcluster)  [unwired: 8 in]
        n90 = call-poly <vilib>:"Read.vi"("error in (no error)"=w401, "Default"=u16 0, "Tag Name"=w394) -> ("error out"=w400:errorcluster, "Value"=→"Min_O2":u16)  [unwired: 7 in]
        n91 = call-poly <vilib>:"Read.vi"("Default"=u16 0, "Tag Name"=w380) -> ("error out"=w374:errorcluster, "Value"=→"Min_N2":u16)  [unwired: 8 in]
        n92 = call-poly <vilib>:"Write.vi"("error in (no error)"=w401, "Value"=w402, "Tag Name"=w387) -> ("error out"=w395:errorcluster)  [unwired: 8 in]
        n93 = call-poly <vilib>:"Read.vi"("error in (no error)"=w400, "Default"=u16 0, "Tag Name"=w387) -> ("error out"=w392:errorcluster, "Value"=→"Max_O2":u16)  [unwired: 7 in]
        n94 = call-poly <vilib>:"Read.vi"("Tag Name"=w317) -> ("error out"=w319:errorcluster, "Value"=→"Temp_Max":u16)  [unwired: 9 in]
        n95 = call-poly <vilib>:"Read.vi"("error in (no error)"=w374, "Default"=u16 0, "Tag Name"=w376) -> ("error out"=w367:errorcluster, "Value"=→"Max_N2":u16)  [unwired: 7 in]
        n96 = call-poly <vilib>:"Write.vi"("error in (no error)"=w395, "Value"=w396, "Tag Name"=w386) -> ()  [unwired: 8 in, 1 out]
        n97 = call-poly <vilib>:"Read.vi"("error in (no error)"=w319, "Tag Name"=w318) -> ("error out"=w296:errorcluster, "Value"=→"Temp_Min 2":u16)  [unwired: 8 in]
        n98 = call-poly <vilib>:"Read.vi"("error in (no error)"=w296, "Tag Name"=w300) -> ("error out"=w295:errorcluster, "Value"=→"Hum_Min":u16)  [unwired: 8 in]
        n99 = call-poly <vilib>:"Read.vi"("error in (no error)"=w295, "Tag Name"=w299) -> ("error out"=w306:errorcluster, "Value"=→"Hum_Max":u16)  [unwired: 8 in]
        n100 = call-poly <vilib>:"Read.vi"("error in (no error)"=w306, "Tag Name"=w298) -> ("error out"=w268:errorcluster, "Value"=→"Hum_Value":u16)  [unwired: 8 in]
        n101 = call-poly <vilib>:"Read.vi"("error in (no error)"=w268, "Default"=u16 0, "Tag Name"=w284) -> ("error out"=w291:errorcluster, "Value"=→"Spare AI-1_Min":u16)  [unwired: 7 in]
        n102 = call-poly <vilib>:"Read.vi"("error in (no error)"=w291, "Default"=u16 0, "Tag Name"=w282) -> ("error out"=w292:errorcluster, "Value"=→"Spare AI-1_Max":u16)  [unwired: 7 in]
        n103 = call-poly <vilib>:"Read.vi"("error in (no error)"=w292, "Default"=u16 0, "Tag Name"=w281) -> ("error out"=w260:errorcluster, "Value"=→"Spare AI-1_Value":u16)  [unwired: 7 in]
        n104 = call-poly <vilib>:"Read.vi"("error in (no error)"=w260, "Tag Name"=w262) -> ("error out"=w269:errorcluster, "Value"=→"Spare AI-2_Min":u16)  [unwired: 8 in]
        n105 = call-poly <vilib>:"Read.vi"("error in (no error)"=w269, "Tag Name"=w264) -> ("error out"=w270:errorcluster, "Value"=→"Spare AI-2_Max":u16)  [unwired: 8 in]
        n106 = call-poly <vilib>:"Read.vi"("error in (no error)"=w270, "Tag Name"=w263) -> ("error out"=w259:errorcluster, "Value"=→"Spare AI-2_Value":u16)  [unwired: 8 in]
        n107 = call-poly <vilib>:"Read.vi"("error in (no error)"=w367, "Default"=u16 0, "Tag Name"=w371) -> ("error out"=w355:errorcluster, "Value"=→"Value_N2":u16)  [unwired: 7 in]
        n108 = call-poly <vilib>:"Read.vi"("error in (no error)"=w355, "Tag Name"=w356) -> ("error out"=w354:errorcluster, "Value"=→"Vel_Min":u16)  [unwired: 8 in]
        n109 = call-poly <vilib>:"Read.vi"("error in (no error)"=w354, "Tag Name"=w353) -> ("error out"=w352:errorcluster, "Value"=→"Vel_Max":u16)  [unwired: 8 in]
        n110 = call-poly <vilib>:"Read.vi"("error in (no error)"=w352, "Tag Name"=w351) -> ("error out"=w338:errorcluster, "Value"=→"Vel_Value":u16)  [unwired: 8 in]
        n111 = call-poly <vilib>:"Read.vi"("error in (no error)"=w338, "Tag Name"=w337) -> ("error out"=w335:errorcluster, "Value"=→"N2 Gas Pressure 1_Min":u16)  [unwired: 8 in]
        n112 = call-poly <vilib>:"Read.vi"("error in (no error)"=w335, "Tag Name"=w336) -> ("error out"=w332:errorcluster, "Value"=→"N2 Gas Pressure 1_Max":u16)  [unwired: 8 in]
        n113 = call-poly <vilib>:"Read.vi"("error in (no error)"=w332, "Tag Name"=w331) -> ("error out"=w316:errorcluster, "Value"=→"N2 Gas Pressure 1_Value":u16)  [unwired: 8 in]
        n114 = call-poly <vilib>:"Read.vi"("error in (no error)"=w316, "Tag Name"=w315) -> ("Value"=→"Temp_Min":u16)  [unwired: 8 in, 1 out]
        n115 = call-poly <vilib>:"Read.vi"("error in (no error)"=w392, "Default"=u16 0, "Tag Name"=w386) -> ("error out"=w381:errorcluster, "Value"=→"Value_O2":u16)  [unwired: 7 in]
        n116 = call-poly <vilib>:"Write.vi"("error in (no error)"=w381, "Value"=w382, "Tag Name"=w380) -> ("error out"=w375:errorcluster)  [unwired: 8 in]
        n117 = call-poly <vilib>:"Write.vi"("error in (no error)"=w375, "Value"=w377, "Tag Name"=w376) -> ("error out"=w372:errorcluster)  [unwired: 8 in]
        n118 = call-poly <vilib>:"Write.vi"("error in (no error)"=w372, "Value"=w369, "Tag Name"=w371) -> ("error out"=w362:errorcluster)  [unwired: 8 in]
        n119 = call-poly <vilib>:"Write.vi"("error in (no error)"=w362, "Value"=w361, "Tag Name"=w356) -> ("error out"=w358:errorcluster)  [unwired: 8 in]
        n120 = call-poly <vilib>:"Write.vi"("error in (no error)"=w358, "Value"=w360, "Tag Name"=w353) -> ("error out"=w357:errorcluster)  [unwired: 8 in]
        n121 = call-poly <vilib>:"Write.vi"("error in (no error)"=w357, "Value"=w359, "Tag Name"=w351) -> ("error out"=w341:errorcluster)  [unwired: 8 in]
        n122 = call-poly <vilib>:"Write.vi"("error in (no error)"=w341, "Value"=w344, "Tag Name"=w337) -> ("error out"=w340:errorcluster)  [unwired: 8 in]
        n123 = call-poly <vilib>:"Write.vi"("error in (no error)"=w340, "Value"=w343, "Tag Name"=w336) -> ("error out"=w339:errorcluster)  [unwired: 8 in]
        n124 = call-poly <vilib>:"Write.vi"("error in (no error)"=w339, "Value"=w342, "Tag Name"=w331) -> ("error out"=w323:errorcluster)  [unwired: 8 in]
        n125 = call-poly <vilib>:"Write.vi"("error in (no error)"=w323, "Value"=w326, "Tag Name"=w315) -> ("error out"=w322:errorcluster)  [unwired: 8 in]
        n126 = call-poly <vilib>:"Write.vi"("error in (no error)"=w322, "Value"=w325, "Tag Name"=w317) -> ("error out"=w321:errorcluster)  [unwired: 8 in]
        n127 = call-poly <vilib>:"Write.vi"("error in (no error)"=w321, "Value"=w324, "Tag Name"=w318) -> ("error out"=w297:errorcluster)  [unwired: 8 in]
        n128 = call-poly <vilib>:"Write.vi"("error in (no error)"=w297, "Value"=w303, "Tag Name"=w300) -> ("error out"=w309:errorcluster)  [unwired: 8 in]
        n129 = call-poly <vilib>:"Write.vi"("error in (no error)"=w309, "Value"=w302, "Tag Name"=w299) -> ("error out"=w308:errorcluster)  [unwired: 8 in]
        n130 = call-poly <vilib>:"Write.vi"("error in (no error)"=w308, "Value"=w301, "Tag Name"=w298) -> ("error out"=w283:errorcluster)  [unwired: 8 in]
        n131 = call-poly <vilib>:"Write.vi"("error in (no error)"=w283, "Value"=w287, "Tag Name"=w284) -> ("error out"=w294:errorcluster)  [unwired: 8 in]
        n132 = call-poly <vilib>:"Write.vi"("error in (no error)"=w294, "Value"=w286, "Tag Name"=w282) -> ("error out"=w293:errorcluster)  [unwired: 8 in]
        n133 = call-poly <vilib>:"Write.vi"("error in (no error)"=w293, "Value"=w285, "Tag Name"=w281) -> ("error out"=w261:errorcluster)  [unwired: 8 in]
        n134 = call-poly <vilib>:"Write.vi"("error in (no error)"=w261, "Value"=w267, "Tag Name"=w262) -> ("error out"=w271:errorcluster)  [unwired: 8 in]
        n135 = call-poly <vilib>:"Write.vi"("error in (no error)"=w271, "Value"=w266, "Tag Name"=w264) -> ("error out"=w257:errorcluster)  [unwired: 8 in]
        n136 = call-poly <vilib>:"Write.vi"("error in (no error)"=w257, "Value"=w265, "Tag Name"=w263) -> ()  [unwired: 8 in, 1 out]
        n137 = Unbundle By Name(w259) -> ("status"=w389:bool)
        n138 = Or(x=w389, y="stop  3") -> (x .or. y?=w388:bool)
      }
      frame #3 {
        w419 = "Value_14" ("Tag Name")
        w420 = "Value_13" ("Tag Name")
        w434 = "Value_12" ("Tag Name")
        w435 = "Value_11" ("Tag Name")
        w436 = "Value_10" ("Tag Name")
        w437 = "Value_9" ("Tag Name")
        w454 = "Value_8" ("Tag Name")
        w459 = "Value_7" ("Tag Name")
        w464 = "Value_6" ("Tag Name")
        w471 = "Value_5" ("Tag Name")
        w477 = "Value_4" ("Tag Name")
        w483 = "Value_3" ("Tag Name")
        w486 = "Value_2" ("Tag Name")
        w496 = "Value_1" ("Tag Name")
        n139 = call-poly <vilib>:"Read.vi"("Tag Name"=w420) -> ("error out"=w418:errorcluster, "Value"=→"Value_13":bool)  [unwired: 9 in]
        n140 = call-poly <vilib>:"Read.vi"("error in (no error)"=w418, "Tag Name"=w419) -> ("error out"=w417:errorcluster, "Value"=→"Value_14":bool)  [unwired: 8 in]
        n141 = call "Read Discrete Inputs.vi"("error in (no error)"=w409, "quantity"=u16 14 ("Quantity"), "starting address"=u16 17 ("Starting Address"), "MB session in"=w412) -> ("error out"=w408:errorcluster, "Inputs"=w411:bool[], "MB session out"=w410:refnum<class "MB_Master_Serial.lvclass">)  [unwired: 5 in]
        n142 = Index Array(array=w411, index=2) -> (element=w481:bool)
        n143 = Index Array(array=w411, index=3) -> (element=w475:bool)
        n144 = Index Array(array=w411, index=4) -> (element=w472:bool)
        n145 = Index Array(array=w411, index=5) -> (element=w466:bool)
        n146 = Index Array(array=w411, index=6) -> (element=w460:bool)
        n147 = Index Array(array=w411, index=7) -> (element=w453:bool)
        n148 = Index Array(array=w411, index=0) -> (element=w497:bool)
        n149 = Index Array(array=w411, index=1) -> (element=w489:bool)
        n150 = Index Array(array=w411, index=8) -> (element=w441:bool)
        n151 = Index Array(array=w411, index=9) -> (element=w440:bool)
        n152 = Index Array(array=w411, index=10) -> (element=w439:bool)
        n153 = Index Array(array=w411, index=11) -> (element=w438:bool)
        n154 = Index Array(array=w411, index=12) -> (element=w424:bool)
        n155 = Index Array(array=w411, index=13) -> (element=w423:bool)
        n156 = call-poly <vilib>:"Write.vi"("error in (no error)"=w408, "Value"=w497, "Tag Name"=w496) -> ("error out"=w490:errorcluster)  [unwired: 8 in]
        n157 = call-poly <vilib>:"Write.vi"("error in (no error)"=w490, "Value"=w489, "Tag Name"=w486) -> ("error out"=w485:errorcluster)  [unwired: 8 in]
        n158 = call-poly <vilib>:"Write.vi"("error in (no error)"=w485, "Value"=w481, "Tag Name"=w483) -> ("error out"=w478:errorcluster)  [unwired: 8 in]
        n159 = call-poly <vilib>:"Write.vi"("error in (no error)"=w478, "Value"=w475, "Tag Name"=w477) -> ("error out"=w469:errorcluster)  [unwired: 8 in]
        n160 = call-poly <vilib>:"Write.vi"("error in (no error)"=w469, "Value"=w472, "Tag Name"=w471) -> ("error out"=w465:errorcluster)  [unwired: 8 in]
        n161 = call-poly <vilib>:"Write.vi"("error in (no error)"=w465, "Value"=w466, "Tag Name"=w464) -> ("error out"=w457:errorcluster)  [unwired: 8 in]
        n162 = call-poly <vilib>:"Write.vi"("error in (no error)"=w457, "Value"=w460, "Tag Name"=w459) -> ("error out"=w451:errorcluster)  [unwired: 8 in]
        n163 = call-poly <vilib>:"Write.vi"("error in (no error)"=w451, "Value"=w453, "Tag Name"=w454) -> ("error out"=w445:errorcluster)  [unwired: 8 in]
        n164 = call-poly <vilib>:"Write.vi"("error in (no error)"=w445, "Value"=w441, "Tag Name"=w437) -> ("error out"=w444:errorcluster)  [unwired: 8 in]
        n165 = call-poly <vilib>:"Write.vi"("error in (no error)"=w444, "Value"=w440, "Tag Name"=w436) -> ("error out"=w443:errorcluster)  [unwired: 8 in]
        n166 = call-poly <vilib>:"Write.vi"("error in (no error)"=w443, "Value"=w439, "Tag Name"=w435) -> ("error out"=w442:errorcluster)  [unwired: 8 in]
        n167 = call-poly <vilib>:"Write.vi"("error in (no error)"=w442, "Value"=w438, "Tag Name"=w434) -> ("error out"=w422:errorcluster)  [unwired: 8 in]
        n168 = call-poly <vilib>:"Write.vi"("error in (no error)"=w422, "Value"=w424, "Tag Name"=w420) -> ("error out"=w421:errorcluster)  [unwired: 8 in]
        n169 = call-poly <vilib>:"Write.vi"("error in (no error)"=w421, "Value"=w423, "Tag Name"=w419) -> ()  [unwired: 8 in, 1 out]
        n170 = call-poly <vilib>:"Read.vi"("error in (no error)"=w490, "Tag Name"=w496) -> ("error out"=w488:errorcluster, "Value"=→"Value_1":bool)  [unwired: 8 in]
        n171 = call-poly <vilib>:"Read.vi"("error in (no error)"=w488, "Tag Name"=w486) -> ("error out"=w484:errorcluster, "Value"=→"Value_2":bool)  [unwired: 8 in]
        n172 = call-poly <vilib>:"Read.vi"("error in (no error)"=w484, "Tag Name"=w483) -> ("error out"=w479:errorcluster, "Value"=→"Value_3":bool)  [unwired: 8 in]
        n173 = call-poly <vilib>:"Read.vi"("error in (no error)"=w479, "Tag Name"=w477) -> ("error out"=w470:errorcluster, "Value"=→"Value_4":bool)  [unwired: 8 in]
        n174 = call-poly <vilib>:"Read.vi"("error in (no error)"=w470, "Tag Name"=w471) -> ("error out"=w463:errorcluster, "Value"=→"Value_5":bool)  [unwired: 8 in]
        n175 = call-poly <vilib>:"Read.vi"("error in (no error)"=w463, "Tag Name"=w464) -> ("error out"=w458:errorcluster, "Value"=→"Value_6":bool)  [unwired: 8 in]
        n176 = call-poly <vilib>:"Read.vi"("error in (no error)"=w458, "Tag Name"=w459) -> ("error out"=w450:errorcluster, "Value"=→"Value_7":bool)  [unwired: 8 in]
        n177 = call-poly <vilib>:"Read.vi"("error in (no error)"=w450, "Tag Name"=w454) -> ("error out"=w433:errorcluster, "Value"=→"Value_8" →"Value_9":bool)  [unwired: 8 in]
        n178 = call-poly <vilib>:"Read.vi"("error in (no error)"=w433, "Tag Name"=w437) -> ("error out"=w432:errorcluster, "Value"=→"Value_10":bool)  [unwired: 8 in]
        n179 = call-poly <vilib>:"Read.vi"("error in (no error)"=w432, "Tag Name"=w436) -> ("error out"=w431:errorcluster)  [unwired: 8 in, 1 out]
        n180 = call-poly <vilib>:"Read.vi"("error in (no error)"=w431, "Tag Name"=w435) -> ("error out"=w430:errorcluster, "Value"=→"Value_11":bool)  [unwired: 8 in]
        n181 = call-poly <vilib>:"Read.vi"("error in (no error)"=w430, "Tag Name"=w434) -> ("Value"=→"Value_12":bool)  [unwired: 8 in, 1 out]
        n182 = Unbundle By Name(w417) -> ("status"=w493:bool)
        n183 = Or(x=w493, y="stop  4") -> (x .or. y?=w492:bool)
      }
      frame #4 {
        w510 = "RH_H2" ("Tag Name")
        w511 = "RH_H1" ("Tag Name")
        w512 = "RH_L2" ("Tag Name")
        w513 = "RH_L1" ("Tag Name")
        w527 = "Temp_H2" ("Tag Name")
        w528 = "Temp_H1" ("Tag Name")
        w529 = "Temp_L2" ("Tag Name")
        w535 = "Temp_L1" ("Tag Name")
        w540 = "N22_H2" ("Tag Name")
        w541 = "N22_H1" ("Tag Name")
        w542 = "N22_L2" ("Tag Name")
        w543 = "N22_L1" ("Tag Name")
        w559 = "Vel_H2" ("Tag Name")
        w560 = "Vel_H1" ("Tag Name")
        w561 = "Vel_L2" ("Tag Name")
        w562 = "Vel_L1" ("Tag Name")
        w571 = "N21_H2" ("Tag Name")
        w572 = "N21_H1" ("Tag Name")
        w573 = "N21_L2" ("Tag Name")
        w574 = "N21_L1" ("Tag Name")
        w628 = "O2_H2" ("Tag Name")
        w631 = "O2_H1" ("Tag Name")
        w623 = "O2_L2" ("Tag Name")
        w639 = "O2_L1" ("Tag Name")
        n184 = call-poly <vilib>:"Read.vi"("Tag Name"=w639) -> ("error out"=w637:errorcluster, "Value"=→"Min_O2 2":u16)  [unwired: 9 in]
        n185 = call-poly <vilib>:"Read.vi"("error in (no error)"=w637, "Tag Name"=w623) -> ("error out"=w630:errorcluster, "Value"=→"Max_O2 2":u16)  [unwired: 8 in]
        n186 = call "Read Input Registers.vi"("error in (no error)"=w505, "quantity"=u16 24 ("Quantity"), "starting address"=u16 100 ("Starting Address"), "MB session in"=w501) -> ("error out"=w504:errorcluster, "Registers"=w502:u16[], "MB session out"=w503:refnum<class "MB_Master_Serial.lvclass">)  [unwired: 5 in]
        n187 = Index Array(array=w502, index #1=0 ("index"), index #2=1 ("index"), index #3=2 ("index"), index #4=3 ("index")) -> (element #1=w643:u16, element #2=w642:u16, element #3=w641:u16, element #4=w640:u16)
        n188 = Index Array(array=w502, index #1=8 ("index"), index #2=9 ("index"), index #3=10 ("index"), index #4=11 ("index")) -> (element #1=w610:u16, element #2=w609:u16, element #3=w608:u16, element #4=w607:u16)
        n189 = Index Array(array=w502, index #1=12 ("index"), index #2=13 ("index"), index #3=14 ("index"), index #4=15 ("index")) -> (element #1=w602:u16, element #2=w601:u16, element #3=w600:u16, element #4=w599:u16)
        n190 = Index Array(array=w502, index #1=16 ("index"), index #2=17 ("index"), index #3=18 ("index"), index #4=19 ("index")) -> (element #1=w594:u16, element #2=w593:u16, element #3=w592:u16, element #4=w591:u16)
        n191 = Index Array(array=w502, index #1=4 ("index"), index #2=5 ("index"), index #3=6 ("index"), index #4=7 ("index")) -> (element #1=w618:u16, element #2=w617:u16, element #3=w616:u16, element #4=w615:u16)
        n192 = Index Array(array=w502, index #1=20 ("index"), index #2=21 ("index"), index #3=22 ("index"), index #4=23 ("index")) -> (element #1=w586:u16, element #2=w585:u16, element #3=w584:u16, element #4=w583:u16)
        n193 = call-poly <vilib>:"Write.vi"("error in (no error)"=w504, "Value"=w643, "Tag Name"=w639) -> ("error out"=w638:errorcluster)  [unwired: 8 in]
        n194 = call-poly <vilib>:"Write.vi"("Value"=w610, "Tag Name"=w562) -> ("error out"=w565:errorcluster)  [unwired: 9 in]
        n195 = call-poly <vilib>:"Write.vi"("error in (no error)"=w638, "Value"=w642, "Tag Name"=w623) -> ("error out"=w636:errorcluster)  [unwired: 8 in]
        n196 = call-poly <vilib>:"Write.vi"("error in (no error)"=w565, "Value"=w609, "Tag Name"=w561) -> ("error out"=w564:errorcluster)  [unwired: 8 in]
        n197 = call-poly <vilib>:"Write.vi"("error in (no error)"=w636, "Value"=w641, "Tag Name"=w631) -> ("error out"=w635:errorcluster)  [unwired: 8 in]
        n198 = call-poly <vilib>:"Read.vi"("error in (no error)"=w630, "Tag Name"=w631) -> ("error out"=w629:errorcluster, "Value"=→"Value_O2 2":u16)  [unwired: 8 in]
        n199 = call-poly <vilib>:"Read.vi"("Tag Name"=w529) -> ("Value"=→"Temp_Max 2":u16)  [unwired: 9 in, 1 out]
        n200 = call-poly <vilib>:"Write.vi"("error in (no error)"=w564, "Value"=w608, "Tag Name"=w560) -> ("error out"=w563:errorcluster)  [unwired: 8 in]
        n201 = call-poly <vilib>:"Write.vi"("error in (no error)"=w635, "Value"=w640, "Tag Name"=w628) -> ("error out"=w582:errorcluster)  [unwired: 8 in]
        n202 = call-poly <vilib>:"Write.vi"("error in (no error)"=w582, "Value"=w618, "Tag Name"=w574) -> ("error out"=w581:errorcluster)  [unwired: 8 in]
        n203 = call-poly <vilib>:"Write.vi"("error in (no error)"=w581, "Value"=w617, "Tag Name"=w573) -> ("error out"=w580:errorcluster)  [unwired: 8 in]
        n204 = call-poly <vilib>:"Write.vi"("error in (no error)"=w580, "Value"=w616, "Tag Name"=w572) -> ("error out"=w579:errorcluster)  [unwired: 8 in]
        n205 = call-poly <vilib>:"Read.vi"("error in (no error)"=w629, "Tag Name"=w628) -> ("error out"=w578:errorcluster, "Value"=→"Value_O2 3":u16)  [unwired: 8 in]
        n206 = call-poly <vilib>:"Read.vi"("error in (no error)"=w578, "Tag Name"=w574) -> ("error out"=w577:errorcluster, "Value"=→"Min_N2 2":u16)  [unwired: 8 in]
        n207 = call-poly <vilib>:"Read.vi"("error in (no error)"=w577, "Tag Name"=w573) -> ("error out"=w576:errorcluster, "Value"=→"Max_N2 2":u16)  [unwired: 8 in]
        n208 = call-poly <vilib>:"Read.vi"("Tag Name"=w528) -> ("Value"=→"Temp_Min 3":u16)  [unwired: 9 in, 1 out]
        n209 = call-poly <vilib>:"Read.vi"("error in (no error)"=w576, "Tag Name"=w572) -> ("error out"=w575:errorcluster, "Value"=→"Value_N2 2":u16)  [unwired: 8 in]
        n210 = call-poly <vilib>:"Write.vi"("error in (no error)"=w563, "Value"=w607, "Tag Name"=w559) -> ("error out"=w544:errorcluster)  [unwired: 8 in]
        n211 = call-poly <vilib>:"Write.vi"("error in (no error)"=w544, "Value"=w602, "Tag Name"=w543) -> ("error out"=w547:errorcluster)  [unwired: 8 in]
        n212 = call-poly <vilib>:"Write.vi"("error in (no error)"=w547, "Value"=w601, "Tag Name"=w542) -> ("error out"=w546:errorcluster)  [unwired: 8 in]
        n213 = call-poly <vilib>:"Write.vi"("error in (no error)"=w546, "Value"=w600, "Tag Name"=w541) -> ("error out"=w545:errorcluster)  [unwired: 8 in]
        n214 = call-poly <vilib>:"Write.vi"("error in (no error)"=w545, "Value"=w599, "Tag Name"=w540) -> ("error out"=w531:errorcluster)  [unwired: 8 in]
        n215 = call-poly <vilib>:"Write.vi"("error in (no error)"=w531, "Value"=w594, "Tag Name"=w535) -> ("error out"=w534:errorcluster)  [unwired: 8 in]
        n216 = call-poly <vilib>:"Write.vi"("error in (no error)"=w534, "Value"=w593, "Tag Name"=w529) -> ("error out"=w533:errorcluster)  [unwired: 8 in]
        n217 = call-poly <vilib>:"Write.vi"("error in (no error)"=w533, "Value"=w592, "Tag Name"=w528) -> ("error out"=w532:errorcluster)  [unwired: 8 in]
        n218 = call-poly <vilib>:"Write.vi"("error in (no error)"=w532, "Value"=w591, "Tag Name"=w527) -> ("error out"=w522:errorcluster)  [unwired: 8 in]
        n219 = call-poly <vilib>:"Write.vi"("error in (no error)"=w522, "Value"=w586, "Tag Name"=w513) -> ("error out"=w521:errorcluster)  [unwired: 8 in]
        n220 = call-poly <vilib>:"Write.vi"("error in (no error)"=w521, "Value"=w585, "Tag Name"=w512) -> ("error out"=w520:errorcluster)  [unwired: 8 in]
        n221 = call-poly <vilib>:"Write.vi"("error in (no error)"=w520, "Value"=w584, "Tag Name"=w511) -> ("error out"=w519:errorcluster)  [unwired: 8 in]
        n222 = call-poly <vilib>:"Write.vi"("error in (no error)"=w579, "Value"=w615, "Tag Name"=w571) -> ()  [unwired: 8 in, 1 out]
        n223 = call-poly <vilib>:"Write.vi"("error in (no error)"=w519, "Value"=w583, "Tag Name"=w510) -> ()  [unwired: 8 in, 1 out]
        n224 = call-poly <vilib>:"Read.vi"("Tag Name"=w527) -> ("error out"=w518:errorcluster, "Value"=→"Temp_Min 4":u16)  [unwired: 9 in]
        n225 = call-poly <vilib>:"Read.vi"("error in (no error)"=w518, "Tag Name"=w513) -> ("error out"=w517:errorcluster, "Value"=→"Hum_Min 2":u16)  [unwired: 8 in]
        n226 = call-poly <vilib>:"Read.vi"("error in (no error)"=w517, "Tag Name"=w512) -> ("error out"=w516:errorcluster, "Value"=→"Hum_Max 2":u16)  [unwired: 8 in]
        n227 = call-poly <vilib>:"Read.vi"("error in (no error)"=w516, "Tag Name"=w511) -> ("error out"=w515:errorcluster, "Value"=→"Hum_Value  2":u16)  [unwired: 8 in]
        n228 = call-poly <vilib>:"Read.vi"("error in (no error)"=w575, "Tag Name"=w571) -> ("error out"=w566:errorcluster, "Value"=→"Value_N2 3":u16)  [unwired: 8 in]
        n229 = call-poly <vilib>:"Read.vi"("error in (no error)"=w566, "Tag Name"=w562) -> ("error out"=w557:errorcluster, "Value"=→"Vel_Min 2":u16)  [unwired: 8 in]
        n230 = call-poly <vilib>:"Read.vi"("error in (no error)"=w557, "Tag Name"=w561) -> ("error out"=w556:errorcluster, "Value"=→"Vel_Max 2":u16)  [unwired: 8 in]
        n231 = call-poly <vilib>:"Read.vi"("error in (no error)"=w556, "Tag Name"=w560) -> ("error out"=w555:errorcluster, "Value"=→"Vel_Value 2":u16)  [unwired: 8 in]
        n232 = call-poly <vilib>:"Read.vi"("error in (no error)"=w555, "Tag Name"=w559) -> ("error out"=w551:errorcluster, "Value"=→"Vel_Value 3":u16)  [unwired: 8 in]
        n233 = call-poly <vilib>:"Read.vi"("error in (no error)"=w551, "Tag Name"=w543) -> ("error out"=w550:errorcluster, "Value"=→"N2 Gas Pressure 1_Min 2":u16)  [unwired: 8 in]
        n234 = call-poly <vilib>:"Read.vi"("error in (no error)"=w550, "Tag Name"=w542) -> ("error out"=w549:errorcluster, "Value"=→"N2 Gas Pressure 1_Max 2":u16)  [unwired: 8 in]
        n235 = call-poly <vilib>:"Read.vi"("error in (no error)"=w549, "Tag Name"=w541) -> ("error out"=w548:errorcluster, "Value"=→"N2 Gas Pressure 1_Value 2":u16)  [unwired: 8 in]
        n236 = call-poly <vilib>:"Read.vi"("error in (no error)"=w548, "Tag Name"=w540) -> ("error out"=w530:errorcluster, "Value"=→"N2 Gas Pressure 1_Value 3":u16)  [unwired: 8 in]
        n237 = call-poly <vilib>:"Read.vi"("error in (no error)"=w530, "Tag Name"=w535) -> ("Value"=→"Temp_Min 5":u16)  [unwired: 8 in, 1 out]
        n238 = call-poly <vilib>:"Read.vi"("error in (no error)"=w515, "Tag Name"=w510) -> ("error out"=w514:errorcluster, "Value"=→"Hum_Value  3":u16)  [unwired: 8 in]
        n239 = Unbundle By Name(w514) -> ("status"=w625:bool)
        n240 = Or(x="stop  5", y=w625) -> (x .or. y?=w624:bool)
      }
    }
  }
  n241 = call-dynamic "Close Session.vi"("error in (no error)"=w2, "MB_Serial session"=w3) -> ("error out"=→"error out":errorcluster)  [unwired: 9 in]
